vi "02señalizacion 307.vi"(5 "Digitales":T3, 6 "Analogicas":dbl[](array[numeric]), 7 "Config Equipo":T4={"Modelo"="", "IP"="", "Puerto"=0, "Time Out"=0, "Med Princ"=0, "Time sin rx"=60, "Reintento"=60, "Ref PD 2"=200} {"Ref PD 2" max=10000 step=1; "Med Princ" items=["1", "2", "3", "4", "5", "6", "7", "8", "9", "10", "11", "12", "13", "14", "15", "16", "17", "18", "19", "20", "21", "22", "23", "24", "25", "26", "27", "28", "29", "30", "31", "32"]}) -> (0 "output control":T2, 1 "error lectura":bool=TRUE, 2 "Estado 307":string="Estado 0", 3 "Señalizacion":T1)   [LabVIEW 2010]
panel:
  out "Indeterminado":bool
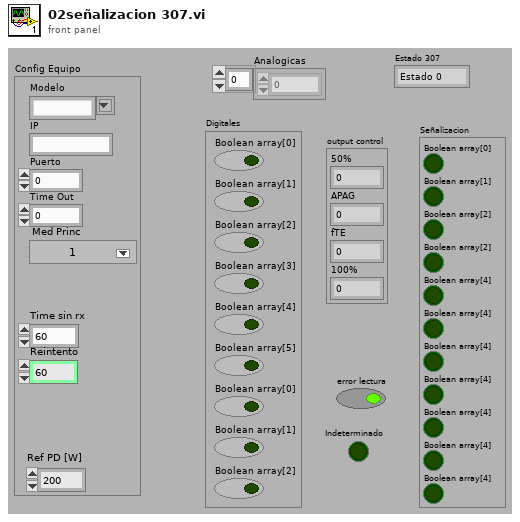
[diagram p1: front panel]
types:
  T1 = cluster{"Boolean array[0]":bool, "Boolean array[1]":bool, "Boolean array[2]":bool, "Boolean array[2]":bool, "Boolean array[4]":bool, "Boolean array[4]":bool, "Boolean array[4]":bool, "Boolean array[4]":bool, "Boolean array[4]":bool, "Boolean array[4]":bool, "Boolean array[4]":bool}
  T2 = cluster{"50%":u8, "APAG":u8, "fTE":u8, "100%":u8}
  T3 = cluster{"Boolean array[0]":bool, "Boolean array[1]":bool, "Boolean array[2]":bool, "Boolean array[3]":bool, "Boolean array[4]":bool, "Boolean array[5]":bool, "Boolean array[0]":bool, "Boolean array[1]":bool, "Boolean array[2]":bool}
  T4 = cluster{"Modelo":string, "IP":string, "Puerto":u16, "Time Out":u16, "Med Princ":u16, "Time sin rx":u16, "Reintento":u16, "Ref PD 2":u16}
  T5 = cluster{"Boolean array[0]":bool, "Boolean array[1]":bool, "Boolean array[2]":bool, "Boolean array[3]":bool, "Boolean array[4]":bool, "Boolean array[5]":bool}
  T6 = cluster{bool, bool, bool, bool, bool, bool, bool, bool, bool, bool, bool}
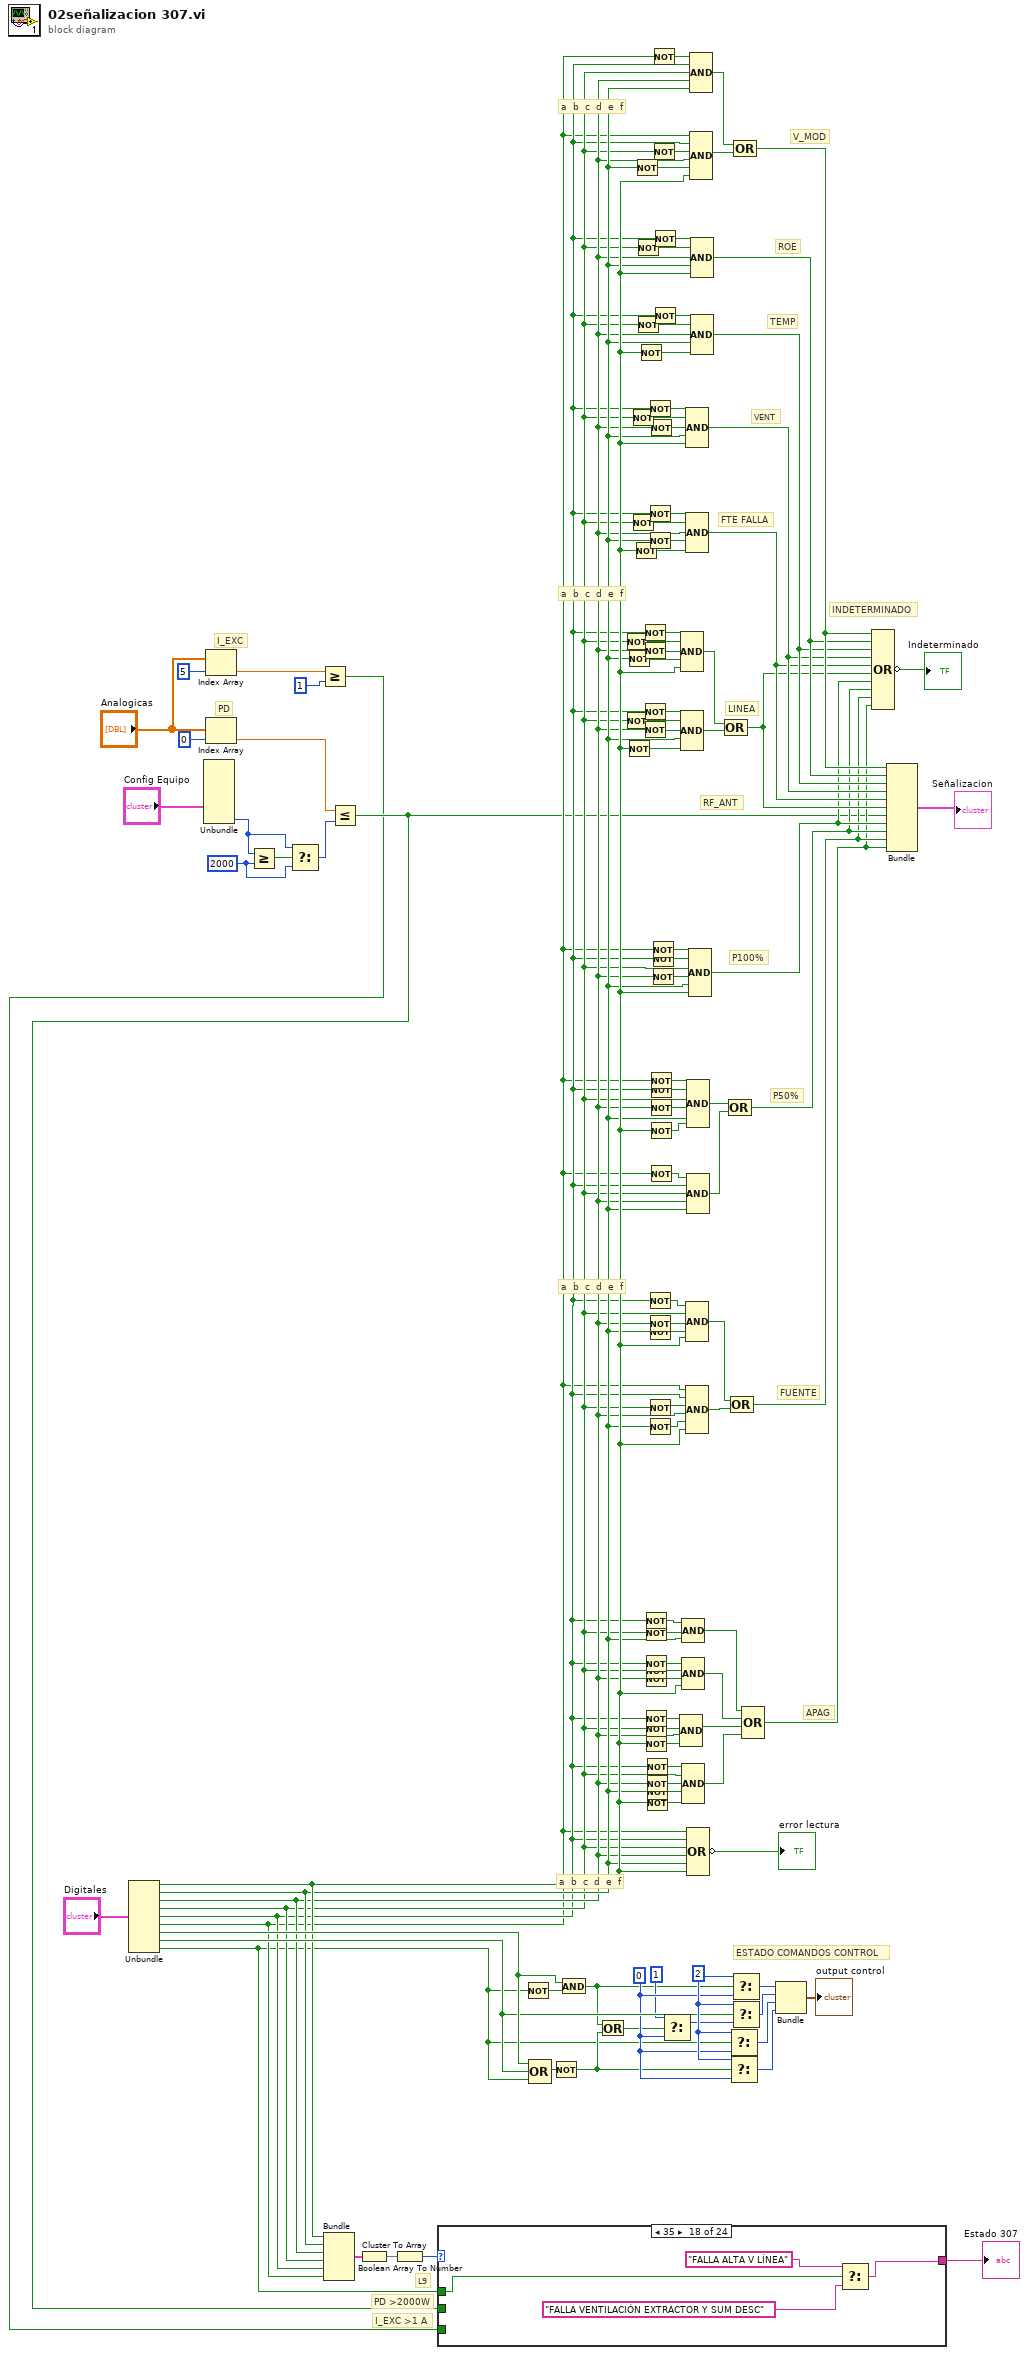
[diagram p0: block diagram]
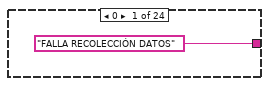
[diagram p2: hidden frame]
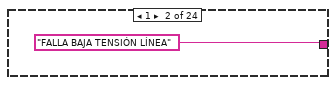
[diagram p3: hidden frame]
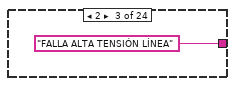
[diagram p4: hidden frame]
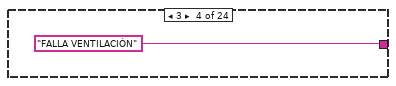
[diagram p5: hidden frame]
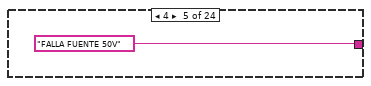
[diagram p6: hidden frame]
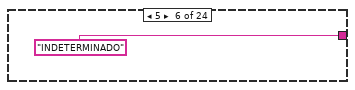
[diagram p7: hidden frame]
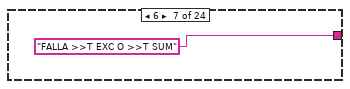
[diagram p8: hidden frame]
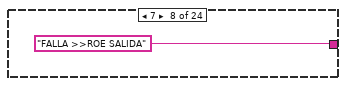
[diagram p9: hidden frame]
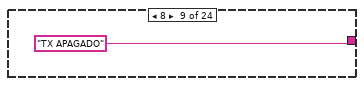
[diagram p10: hidden frame]
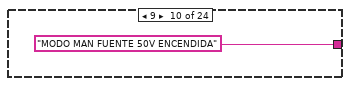
[diagram p11: hidden frame]
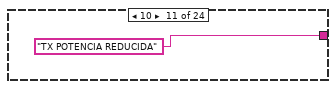
[diagram p12: hidden frame]
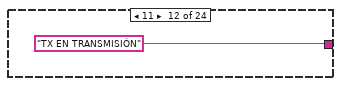
[diagram p13: hidden frame]
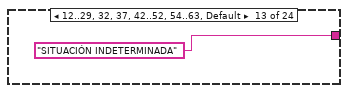
[diagram p14: hidden frame]
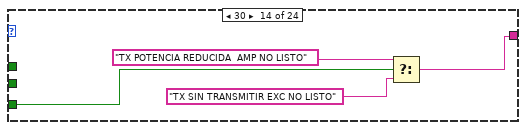
[diagram p15: hidden frame]
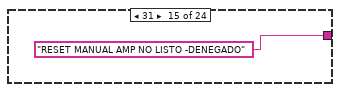
[diagram p16: hidden frame]
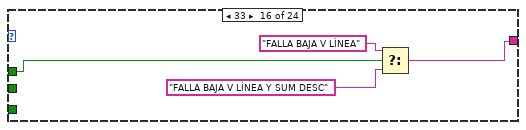
[diagram p17: hidden frame]
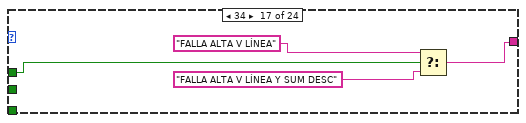
[diagram p18: hidden frame]
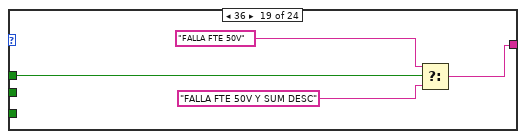
[diagram p19: hidden frame]
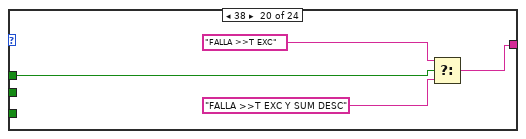
[diagram p20: hidden frame]
diagram:
  w27 = u16 2000 ("y")
  w109 = u8 2 ("f")
  w23 = u8 0 ("f")
  # "I_EXC"
  # "L9"
  # "I_EXC >1 A"
  # "PD >2000W"
  # "a  b  c  d  e  f"
  # "V_MOD"
  # "ROE"
  # "TEMP"
  # "VENT"
  # "a  b  c  d  e  f"
  # "FTE FALLA"
  # "LINEA"
  # "P100%"
  # "P50%"
  # "FUENTE"
  # "a  b  c  d  e  f"
  # "ESTADO COMANDOS CONTROL"
  # "INDETERMINADO"
  # "APAG"
  # "a  b  c  d  e  f"
  # "RF_ANT"
  # "PD"
  n1 = Unbundle("Digitales") -> ("Boolean array[0]"=w17:bool, "Boolean array[1]"=w16:bool, "Boolean array[2]"=w15:bool, "Boolean array[3]"=w14:bool, "Boolean array[4]"=w13:bool, "Boolean array[5]"=w12:bool, "Boolean array[0]"=w107:bool, "Boolean array[1]"=w24:bool, "Boolean array[2]"=w3:bool)
  n2 = Unbundle("Config Equipo") -> ("Ref PD 2"=w28:u16)  [unwired: 7 out]
  n3 = Index Array(array="Analogicas", index=5 ("offset (0)")) -> (element=w9:dbl)
  n4 = Index Array(array="Analogicas", index=0 ("offset (0)")) -> (element=w114:dbl)
  n5 = Greater Or Equal?(x=w28, y=w27) -> (x >= y?=w29:bool)
  n6 = Select(t=w28, s=w29, f=w27) -> (s? t:f=w26:u16)
  n7 = Greater Or Equal?(x=w9, y=u16 1) -> (x >= y?=w1:bool)
  n8 = Bundle("Boolean array[0]"=w17, "Boolean array[1]"=w16, "Boolean array[2]"=w15, "Boolean array[3]"=w14, "Boolean array[4]"=w13, "Boolean array[5]"=w12) -> (w7:T5)  [unwired: 1 in]
  n9 = Less Or Equal?(x=w114, y=w26) -> (x <= y?=w2:bool)
  n10 = Cluster To Array(cluster=w7) -> (array=w6:bool[])
  n11 = Boolean Array To Number(Boolean array=w6) -> (number=w5:u32)
  n12 = case shown="35" w5 {
    tunnel: ["FALLA RECOLECCIÓN DATOS" "FALLA BAJA TENSIÓN LÍNEA" "FALLA ALTA TENSIÓN LÍNEA" "FALLA VENTILACIÓN" "FALLA FUENTE 50V" "INDETERMINADO" "FALLA >>T EXC O >>T SUM" "FALLA >>ROE SALIDA" "TX APAGADO" "MODO MAN FUENTE 50V ENCENDIDA" "TX POTENCIA REDUCIDA" "TX EN TRANSMISIÓN" "SITUACIÓN INDETERMINADA" w128 "RESET MANUAL AMP NO LISTO -DENEGADO" w133 w137 w141 w147 w149 w153 w157 w161 w165] -> w4
    tunnel: w3 -> [_ _ _ _ _ _ _ _ _ _ _ _ _ _ _ w136 w140 w144 w148 w152 w156 w160 w164 w168]
    tunnel: w2 -> [_ _ _ _ _ _ _ _ _ _ _ _ _ _ _ _ _ _ _ _ _ _ _ _]
    tunnel: w1 -> [_ _ _ _ _ _ _ _ _ _ _ _ _ w131 _ _ _ _ _ _ _ _ _ _]
    frame 0 {
    }
    frame 1 {
    }
    frame 2 {
    }
    frame 3 {
    }
    frame 4 {
    }
    frame 5 {
    }
    frame 6 {
    }
    frame 7 {
    }
    frame 8 {
    }
    frame 9 {
    }
    frame 10 {
    }
    frame 11 {
    }
    frame 12..29, 32, 37, 42..52, 54..63, Default {
    }
    frame 30 {
      n13 = Select(t="TX POTENCIA REDUCIDA  AMP NO LISTO", s=w131, f="TX SIN TRANSMITIR EXC NO LISTO") -> (s? t:f=w128:string)
    }
    frame 31 {
    }
    frame 33 {
      n14 = Select(t="FALLA BAJA V LÍNEA", s=w136, f="FALLA BAJA V LÍNEA Y SUM DESC") -> (s? t:f=w133:string)
    }
    frame 34 {
      n15 = Select(t="FALLA ALTA V LÍNEA", s=w140, f="FALLA ALTA V LÍNEA Y SUM DESC") -> (s? t:f=w137:string)
    }
    frame 35 {
      n16 = Select(t="FALLA ALTA V LÍNEA", s=w144, f="FALLA VENTILACIÓN EXTRACTOR Y SUM DESC") -> (s? t:f=w141:string)
    }
    frame 36 {
      n17 = Select(t="FALLA FTE 50V", s=w148, f="FALLA FTE 50V Y SUM DESC") -> (s? t:f=w147:string)
    }
    frame 38 {
      n18 = Select(t="FALLA >>T EXC", s=w152, f="FALLA >>T EXC Y SUM DESC") -> (s? t:f=w149:string)
    }
    frame 39 {
      n19 = Select(t="FALLA >>ROE SALIDA", s=w156, f="FALLA >>ROE SALIDA Y SUM DESC") -> (s? t:f=w153:string)
    }
    frame 40 {
      n20 = Select(t="TX APAGADO", s=w160, f="TX APAGADO Y SUM DESC") -> (s? t:f=w157:string)
    }
    frame 41 {
      n21 = Select(t="FUENTE 50V ENCENDIDA", s=w164, f="MODO MAN FTE50V SIN RF POR SUM DESC") -> (s? t:f=w161:string)
    }
    frame 53 {
      n22 = Select(t="MODO TLCM FTE50V ENCENDIDA", s=w168, f="FTE50V SIN RF POR SUM DESC") -> (s? t:f=w165:string)
    }
  }
  "Estado 307" <- w4
  n23 = Not(x=w3) -> (.not. x?=w108:bool)
  n24 = Compound Arithmetic op=OR(w107, w24, w3) -> (w110:bool)
  n25 = Not(x=w110) -> (.not. x?=w19:bool)
  n26 = And(x=w107, y=w108) -> (x .and. y?=w18:bool)
  n27 = Or(x=w18, y=w19) -> (x .or. y?=w20:bool)
  n28 = Not(x=w14) -> (.not. x?=w68:bool)
  n29 = Not(x=w14) -> (.not. x?=w64:bool)
  n30 = Not(x=w16) -> (.not. x?=w59:bool)
  n31 = Not(x=w17) -> (.not. x?=w62:bool)
  n32 = Not(x=w14) -> (.not. x?=w54:bool)
  n33 = Not(x=w14) -> (.not. x?=w57:bool)
  n34 = Not(x=w17) -> (.not. x?=w55:bool)
  n35 = Not(x=w16) -> (.not. x?=w42:bool)
  n36 = Not(x=w14) -> (.not. x?=w47:bool)
  n37 = Not(x=w14) -> (.not. x?=w50:bool)
  n38 = Not(x=w17) -> (.not. x?=w51:bool)
  n39 = Not(x=w13) -> (.not. x?=w67:bool)
  n40 = Not(x=w15) -> (.not. x?=w60:bool)
  n41 = Not(x=w13) -> (.not. x?=w65:bool)
  n42 = Not(x=w15) -> (.not. x?=w61:bool)
  n43 = Not(x=w13) -> (.not. x?=w100:bool)
  n44 = Not(x=w14) -> (.not. x?=w99:bool)
  n45 = Not(x=w13) -> (.not. x?=w98:bool)
  n46 = Not(x=w14) -> (.not. x?=w97:bool)
  n47 = Not(x=w15) -> (.not. x?=w96:bool)
  n48 = Not(x=w13) -> (.not. x?=w95:bool)
  n49 = Not(x=w14) -> (.not. x?=w94:bool)
  n50 = Not(x=w17) -> (.not. x?=w93:bool)
  n51 = Not(x=w13) -> (.not. x?=w92:bool)
  n52 = Not(x=w15) -> (.not. x?=w91:bool)
  n53 = Not(x=w16) -> (.not. x?=w90:bool)
  n54 = Not(x=w17) -> (.not. x?=w89:bool)
  n55 = Not(x=w13) -> (.not. x?=w53:bool)
  n56 = Not(x=w13) -> (.not. x?=w58:bool)
  n57 = Not(x=w16) -> (.not. x?=w56:bool)
  n58 = Not(x=w13) -> (.not. x?=w81:bool)
  n59 = Not(x=w15) -> (.not. x?=w84:bool)
  n60 = Not(x=w16) -> (.not. x?=w83:bool)
  n61 = Not(x=w14) -> (.not. x?=w25:bool)
  n62 = Not(x=w16) -> (.not. x?=w82:bool)
  n63 = Not(x=w15) -> (.not. x?=w52:bool)
  n64 = Not(x=w12) -> (.not. x?=w75:bool)
  n65 = Not(x=w13) -> (.not. x?=w74:bool)
  n66 = Not(x=w15) -> (.not. x?=w73:bool)
  n67 = Not(x=w17) -> (.not. x?=w76:bool)
  n68 = Not(x=w12) -> (.not. x?=w72:bool)
  n69 = Not(x=w12) -> (.not. x?=w69:bool)
  n70 = Not(x=w13) -> (.not. x?=w70:bool)
  n71 = Not(x=w15) -> (.not. x?=w71:bool)
  n72 = Not(x=w12) -> (.not. x?=w46:bool)
  n73 = Not(x=w14) -> (.not. x?=w43:bool)
  n74 = Not(x=w13) -> (.not. x?=w48:bool)
  n75 = Not(x=w13) -> (.not. x?=w49:bool)
  n76 = Select(t=u8 1, s=w20, f=w23) -> (s? t:f=w22:u8)
  n77 = Compound Arithmetic op=AND(w95, w94, w15, w93) -> (w87:bool)
  n78 = Compound Arithmetic op=AND(w67, w68, w60, w59, w17) -> (w66:bool)
  n79 = Compound Arithmetic op=AND(w65, w64, w61, w16, w62) -> (w63:bool)
  n80 = Compound Arithmetic op=AND(w100, w99, w16) -> (w85:bool)
  n81 = Compound Arithmetic op=AND(w98, w97, w96, w17) -> (w86:bool)
  n82 = Compound Arithmetic op=AND(w92, w14, w91, w90, w89) -> (w88:bool)
  n83 = Compound Arithmetic op=AND(w53, w54, w52, w16, w17) -> (w37:bool)
  n84 = Compound Arithmetic op=AND(w58, w57, w15, w56, w55) -> (w36:bool)
  n85 = Compound Arithmetic op=AND(w81, w14, w84, w83, w17) -> (w79:bool)
  n86 = Compound Arithmetic op=AND(w12, w13, w25, w15, w82, w17) -> (w80:bool)
  n87 = Compound Arithmetic op=AND(w75, w74, w14, w73, w16, w76) -> (w77:bool)
  n88 = Compound Arithmetic op=AND(w72, w13, w14, w15, w16) -> (w78:bool)
  n89 = Compound Arithmetic op=OR(w12, w13, w14, w15, w16, w17) -> (invert →"error lectura":bool)
  n90 = Compound Arithmetic op=AND(w69, w70, w14, w71, w16, w17) -> (w34:bool)
  n91 = Compound Arithmetic op=AND(w46, w13, w14, w15, w16) -> (w45:bool)
  n92 = Compound Arithmetic op=AND(w12, w13, w43, w15, w42, w17) -> (w44:bool)
  n93 = Compound Arithmetic op=AND(w48, w47, w15, w16, w17) -> (w39:bool)
  n94 = Compound Arithmetic op=AND(w49, w50, w15, w16, w51) -> (w38:bool)
  n95 = Compound Arithmetic op=OR(w66, w63) -> (w35:bool)
  n96 = Compound Arithmetic op=OR(w77, w78) -> (w33:bool)
  n97 = Select(t=w109, s=w3, f=w23) -> (s? t:f=w104:u8)
  n98 = Select(t=w109, s=w19, f=w23) -> (s? t:f=w103:u8)
  n99 = Compound Arithmetic op=OR(w79, w80) -> (w32:bool)
  n100 = Select(t=w109, s=w18, f=w23) -> (s? t:f=w106:u8)
  n101 = Select(t=w109, s=w24, f=w22) -> (s? t:f=w105:u8)
  n102 = Compound Arithmetic op=OR(w45, w44) -> (w40:bool)
  n103 = Compound Arithmetic op=OR(w85, w86, w87, w88) -> (w31:bool)
  n104 = Bundle("f"=w106, "f"=w105, "f"=w104, "f"=w103) -> (→"output control":cluster{"f":u8, "f":u8, "f":u8, "f":u8})  [unwired: 1 in]
  n105 = Compound Arithmetic op=OR(w40, w39, w38, w37, w36, w35, w34, w33, w32, w31) -> (invert →"Indeterminado":bool)
  n106 = Bundle(w40, w39, w38, w37, w36, w35, w2, w34, w33, w32, w31) -> (→"Señalizacion":T6)  [unwired: 1 in]
